vi "Get System Resources.vi"(8 "error in (no error)":errorcluster) -> (0 "error out":errorcluster, 3 "System Resources":T1)   [LabVIEW 2020]
doc: "This VI gets the System Resources variable from the appropriate notifier."
uses:
  Type Definitions/System Resources.ctl
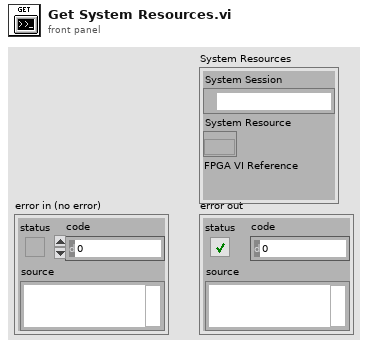
[diagram p1: front panel]
types:
  T1 = typedef "System Resources.ctl" = cluster{"System Session":refnum<k21>, "System Resource":refnum<k20>, "FPGA VI Reference":refnum<k20>}
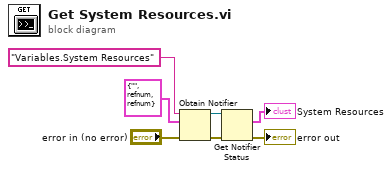
[diagram p0: block diagram]
diagram:
  n1 = Obtain Notifier(name (unnamed)="Variables.System Resources", notification data type=T1 {"System Session"="", "System Resource"=refnum, "FPGA VI Reference"=refnum} ("cluster"), error in (no error)="error in (no error)") -> (notifier out=w5:refnum<notifier>, error out=w4:errorcluster)  [unwired: 1 in, 1 out]
  n2 = Get Notifier Status(notifier=w5, error in (no error)=w4) -> (current notification=→"System Resources":T1, error out=→"error out":errorcluster)  [unwired: 3 out]
